vi "writeNumberOfImagesXML.vi"(8 "error in (no error)":errorcluster, 10 "NativeXML in":refnum<class "NativeXML.lvclass">, 11 "PixelflySettings in":refnum<class "PixelflySettings.lvclass">) -> (0 "error out":errorcluster, 2 "NativeXML out":refnum<class "NativeXML.lvclass">, 3 "PixelflySettings out":refnum<class "PixelflySettings.lvclass">)   [LabVIEW 2011, in "Tools.lvlib" / "Settings.lvlib" / "PixelflySettings.lvclass"]
uses:
  PixelflySettings.lvclass
  NativeXML/NativeXML.lvclass
  PixelflySettings.lvclass/PixelflySettings.ctl
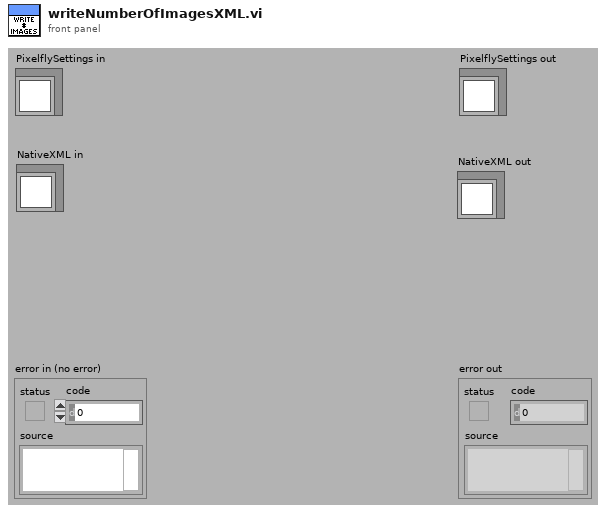
[diagram p1: front panel]
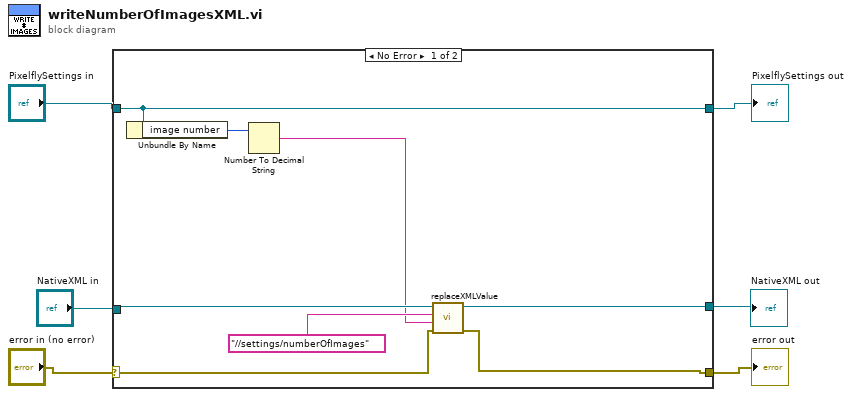
[diagram p0: block diagram]
diagram:
  n1 = case shown="No Error" "error in (no error)" {
    selector: "error in (no error)" -> [w10 w17]
    tunnel: [w9 w17] -> w4
    tunnel: [w14 w16] -> w5
    tunnel: "PixelflySettings in" -> [w14 w16]
    tunnel: "NativeXML in" -> [w13 w15]
    tunnel: [w12 w15] -> w3
    frame No Error {
      n2 = Unbundle By Name(w14) -> ("image number"=w8:i32)
      n3 = Number To Decimal String(number=w8) -> (decimal integer string=w7:string)  [unwired: 1 in]
      n4 = call "replaceXMLValue.vi"("error in (no error)"=w10, "value"=w7, "replace in"="//settings/numberOfImages", "NativeXML in"=w13) -> ("error out"=w9:errorcluster, "NativeXML out"=w12:refnum<class "NativeXML.lvclass">)  [unwired: 6 in]
    }
    frame Error {
    }
  }
  "error out" <- w4
  "PixelflySettings out" <- w5
  "NativeXML out" <- w3
